vi "onAssertionSlippage.vi"(7 "BananaPeel in":refnum<class "BananaPeel.lvclass">, 11 "Leaf.Assertion":refnum<class "Leaf.Assertion.lvclass">) -> (0 "error out":errorcluster, 3 "Leaf.Assertion":refnum<class "Leaf.Assertion.lvclass">)   [LabVIEW 2021, in "Bananas.lvlib" / "BananaPeel.lvclass"]
uses:
  BananaPeel.lvclass
  Leaf.Assertion/Leaf.Assertion.lvclass
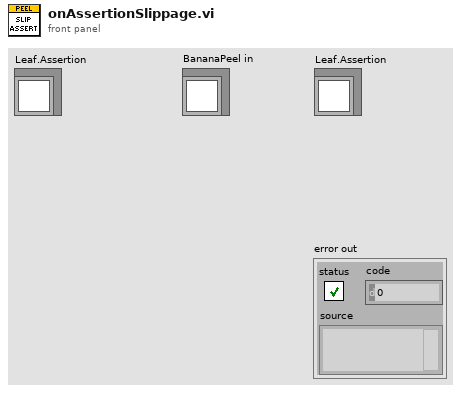
[diagram p1: front panel]
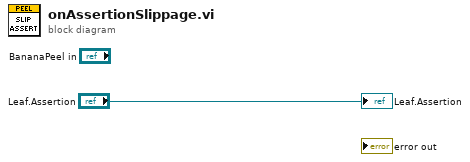
[diagram p0: block diagram]
diagram:
  "Leaf.Assertion" <- "Leaf.Assertion"
